vi "Actor Core.vi"(8 "error in":errorcluster, 11 "XBoxController in":refnum<class "XBoxController.lvclass">) -> (0 "error out":errorcluster, 3 "Actor out":refnum<class "Actor.lvclass">)   [LabVIEW 2013, in "XBoxController.lvclass"]
doc: "(<B>Filename</B>: Actor Framework.lvlib:Actor.lvclass:Actor Core.vi)\n\nReceives messages to the actor, reacts to them, and initiates any error handling that may shut the actor down.\n\nDescendant classes may override this VI to append parallel tasks for the actor to complete while it handles messages. Overrides use the Call Parent Method node."
uses:
  XBoxController.lvclass
  <vilib>/ActorFramework/Actor/Actor.lvclass
  XBoxJoystick.ctl
  XBoxController.lvclass/XBoxController.ctl
  System/System.lvclass
panel:
  out "Right XBoxJoystick":T1 {"Right" scale=-1.0..1.0; "Forward" scale=-1.0..1.0}
  out "Left XBoxJoystick":T1 {"Right" scale=-1.0..1.0; "Forward" scale=-1.0..1.0}
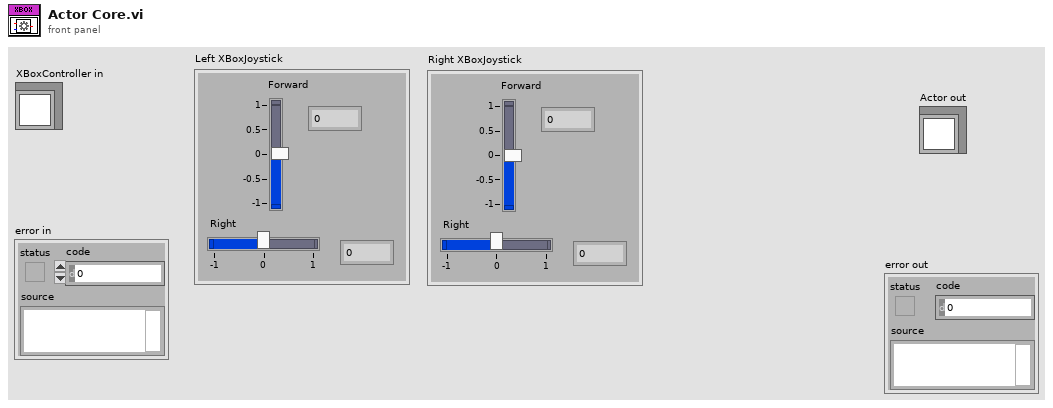
[diagram p1: front panel]
types:
  T1 = typedef "XBoxController.lvclass/XBoxJoystick.ctl" = cluster{"Forward":dbl, "Right":dbl}
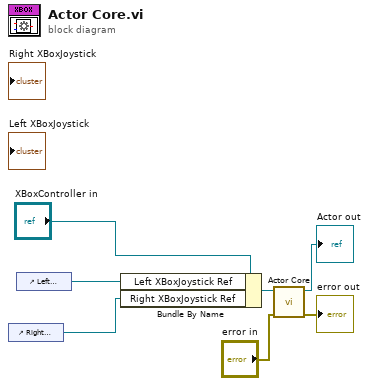
[diagram p0: block diagram]
diagram:
  n1 = control-ref of="Right XBoxJoystick"() -> (w1:refnum<vi>)
  n2 = control-ref of="Left XBoxJoystick"() -> (w2:refnum<vi>)
  n3 = Bundle By Name(cluster="XBoxController in", "Left XBoxJoystick Ref"=w2, "Right XBoxJoystick Ref"=w1) -> (w3:refnum<class "XBoxController.lvclass">)
  n4 = call-parent "Actor Core.vi"("error in"="error in", "Actor in"=w3) -> ("error out"=→"error out":errorcluster, "Actor out"=→"Actor out":refnum<class "Actor.lvclass">)  [unwired: 8 in]
